vi "Add Switch HW Custom Device.vi"(8 "error in (no error)":errorcluster, 10 "Settings":T1, 11 "Target in":refnum<k24>) -> (0 "error out":errorcluster, 2 "Switch HW Custom Device":refnum<k24>, 3 "Target out":refnum<k24>)   [LabVIEW 2017, in "Switch Scripting.lvlib"]
uses:
  Switch Scripting.lvlib
  NationalInstruments.VeriStand.SystemDefinitionAPI
  Switch HW Custom Device Settings.ctl
  Shared/Constants and GUIDs.vi
  Shared/Engine Simulation Toolkit Shared.lvlib
  System Explorer/Engine Simulation Toolkit System Explorer.lvlib
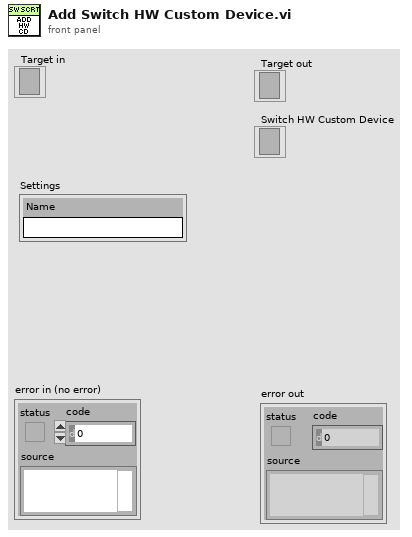
[diagram p1: front panel]
types:
  T1 = typedef "Switch Scripting.lvlib/Switch HW Custom Device Settings.ctl" = cluster{"Name":string}
  T2 = typedef "Custom Device API.lvlib/Custom Device Item Ref.ctl" = u64
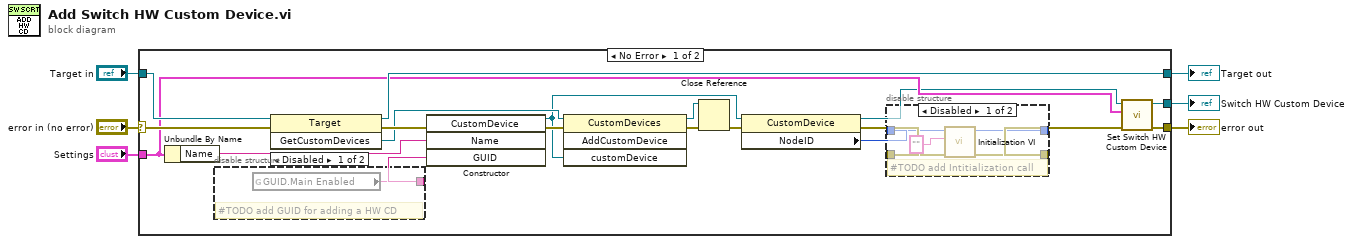
[diagram p0: block diagram]
diagram:
  n1 = case shown="No Error" "error in (no error)" {
    selector: "error in (no error)" -> [w25 w33]
    tunnel: [w15 w33] -> w6
    tunnel: "Target in" -> [w24 w32]
    tunnel: [w19 w32] -> w3
    tunnel: "Settings" -> [w13 _]
    tunnel: [w16 _] -> w1
    frame No Error {
      n2 = Unbundle By Name(w13) -> ("Name"=w14:string)
      n3 = disable-structure shown="Disabled" {
        disable-tunnel: [w31 _] -> w22
        frame Disabled {
          # "#TODO add GUID for adding a HW CD"
          n4 = global read "Constants and GUIDs.vi" "GUID.Main Enabled"() -> (w31:string)
        }
        frame Enabled {
        }
      }
      n5 = invoke class="Target" method="GetCustomDevices"(reference=w24, error in=w25) -> (reference out=w19:refnum<k24>, error out=w23:errorcluster, "GetCustomDevices"=w21:refnum<k24>)  [unwired: 1 in]
      n6 = constructor class="CustomDevice"(error in=w23, "Name"=w14, "GUID"=w22) -> (reference out=w12:refnum<k24>, error out=w20:errorcluster)  [unwired: 2 in, 3 out]
      n7 = invoke class="CustomDevices" method="AddCustomDevice"(reference=w21, error in=w20, "customDevice"=w12) -> (reference out=w18:refnum<k24>, error out=w17:errorcluster)  [unwired: 1 in, 2 out]
      n8 = Close Reference(reference=w18, error in (no error)=w17) -> (error out=w10:errorcluster)
      n9 = property class="CustomDevice"(reference=w12, error in=w10) -> (reference out=w11:refnum<k24>, error out=w9:errorcluster, "NodeID"=w8:u64)
      n10 = disable-structure shown="Disabled" {
        disable-tunnel: w9 -> [w30 _]
        disable-tunnel: w8 -> [w29 _]
        disable-tunnel: [w28 _] -> _
        disable-tunnel: [w27 _] -> w7
        frame Disabled {
          # "#TODO add Intitialization call"
          n11 = call "Initialization VI.vi"("error in (no error)"=w30, "Custom XML"="", "Device Item Ref in"=w29) -> ("error out"=w27:errorcluster, "Device Item Ref out"=w28:T2)  [unwired: 7 in]
        }
        frame Enabled {
        }
      }
      n12 = call "Set Switch HW Custom Device.vi"("error in (no error)"=w7, "Settings"=w13, "Switch HW Custom Device in"=w11) -> ("error out"=w15:errorcluster, "Switch HW Custom Device out"=w16:refnum<k24>)  [unwired: 7 in]
    }
    frame Error {
    }
  }
  "Target out" <- w3
  "error out" <- w6
  "Switch HW Custom Device" <- w1
